vi "4.5.vi"() -> ()   [LabVIEW 2017]
panel:
  out "循环次数":dbl
  in  "指定值":dbl
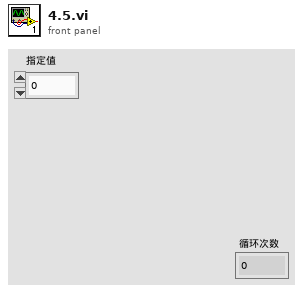
[diagram p1: front panel]
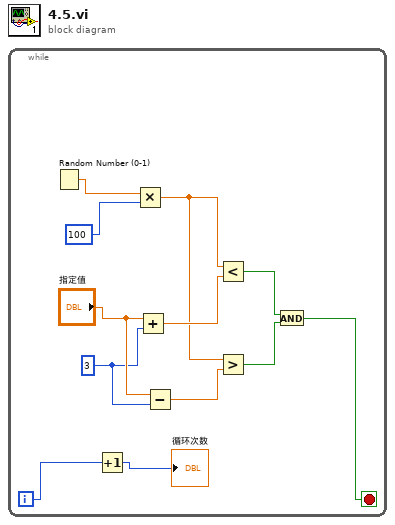
[diagram p0: block diagram]
diagram:
  n1 = while {
    i -> [w2]
    stop <- w4 stop-if-true
    w9 = 3
    n2 = Random Number (0-1)() -> (number: 0 to 1=w1:dbl)
    n3 = Increment(x=w2) -> (x+1=→"循环次数":i32)
    n4 = Multiply(x=w1, y=100) -> (x*y=w8:dbl)
    n5 = Add(x="指定值", y=w9) -> (x+y=w11:dbl)
    n6 = Subtract(x="指定值", y=w9) -> (x-y=w7:dbl)
    n7 = Less?(x=w8, y=w11) -> (x < y?=w6:bool)
    n8 = Greater?(x=w8, y=w7) -> (0:w5:bool)
    n9 = And(x=w6, y=w5) -> (x .and. y?=w4:bool)
  }
